vi "E725_Simple_Test.vi"(0 "System no.":i32=1 min=1 max=4 step=1, 2 "Interface":u16(ring) items=["RS232", "TCP/IP", "USB"], 3 "Timeout":u32=5000, 5 "error in":errorcluster, 6 "RS232 settings":cluster{"Portnumber":u16, "Baudrate":u16}={"Portnumber"=0, "Baudrate"=5} {"Baudrate" items=["9600", "14400", "19200", "38400", "57600", "115200"]; "Portnumber" items=["COM1", "COM2", "COM3", "COM4", "COM5", "COM6", "COM7", "COM8", "COM9"]}, 7 "TCP/IP settings":T1={"Host address/name"="localhost", "Port"=50000, "Board"=0, "TCP/IP Search?"=TRUE}, 8 "USB settings":cluster{"S/N":string, "USB Search?":bool}={"S/N"="", "USB Search?"=TRUE}) -> (14 "Identification":string, 15 "Helpstring":string, 16 "Conn. Axes":string[](array[string]), 17 "Position":dbl[](array[numeric]) format="%.6f", 19 "error out":errorcluster)   [LabVIEW 2009]
doc: "This simple test VI is a stand-alone sample application. Use the Help?Show Context Help menu sequence in the LabVIEW environment to display the Context Help window with the VI and control/indicator descriptions.\n\nSpecify \n¢ System no. (= 1 in a one-system configuration),\n¢ Interface (= RS232, TCP/IP or USB)\n¢ Timeout value (in milliseconds)\n¢ and interface settings first.\n\nThen start the VI. The VI will open a connection to the E-712 and query the controller for its identification string (*IDN?), help string (HLP?), the IDs (SAI?) and stage names (CST?) of the connected axes and their current position values (POS?). The diagram shows how to combine the driver and support VIs for these tasks."
panel:
  out "Stage names":string[](array[string])
  # "Simple E-712 communication test program"
  # "Select E-712 interface, timeout value and interface settings first, then start the VI. \nThe VI will open the chosen port, query for the connected axes (SAI?), the stage names (SAI?), the position (POS?), Identification (*IDN?) and help string\n(HLP?). See VI and control/ indicator information for details."
  # "Only for\nInterface = \nTCP/IP:"
  # "Only for\nInterface = \nRS232:"
  # "Only for\nInterface = \nUSB:"
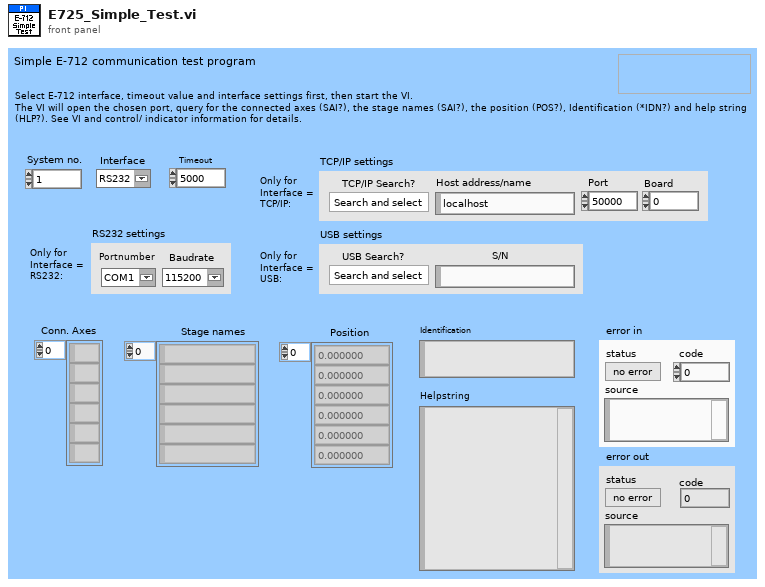
[diagram p1: front panel]
types:
  T1 = cluster{"Host address/name":string, "Port":i32, "Board":i32, "TCP/IP Search?":bool}
  T2 = cluster{"Host address/name":string, "Port":i32, "Board":i32}
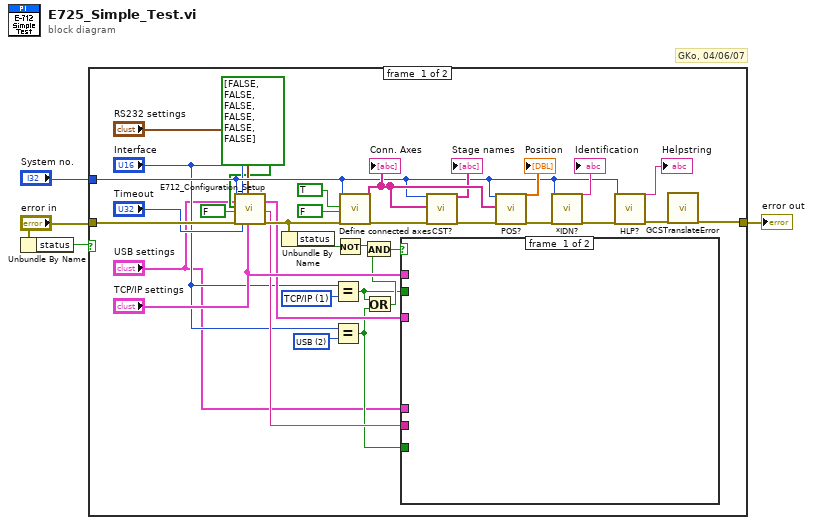
[diagram p0: block diagram]
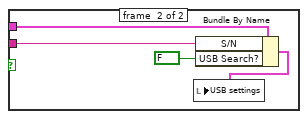
[diagram p3: hidden frame]
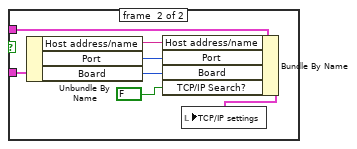
[diagram p4: hidden frame]
diagram:
  # "GKo, 04/06/07"
  n1 = Unbundle By Name("error in") -> ("status"=w2:bool)
  n2 = case shown="False" w2 {
    tunnel: [w37 w55] -> w3
    tunnel: "error in" -> [w24 w55]
    tunnel: "System no." -> [w23 _]
    frame #0 {
      w10 = u16 2 items=["RS232", "TCP/IP", "USB"] ("Interface")
      w11 = u16 1 items=["RS232", "TCP/IP", "USB"] ("Interface")
      n3 = call "E712_Configuration_Setup.vi"("System no."=w23, "USB settings"="USB settings", "Are stages connected?"=bool[] [FALSE, FALSE, FALSE, FALSE, FALSE, FALSE], "Change servo status to ON?"=FALSE ("Connected?"), "error in"=w24, "Interface"="Interface", "Timeout"="Timeout", "RS232 settings"="RS232 settings", "TCP/IP settings"="TCP/IP settings") -> ("TCP/IP settings out"=w14:T2, "USB: S/N out"=w13:string, "error out"=w19:errorcluster)  [unwired: 6 in, 2 out]
      n4 = Unbundle By Name(w19) -> ("status"=w18:bool)
      n5 = Equal?(x="Interface", y=w11) -> (x = y?=w8:bool)
      n6 = Equal?(x="Interface", y=w10) -> (x = y?=w7:bool)
      n7 = Not(x=w18) -> (.not. x?=w16:bool)
      n8 = call "Define connected axes.vi"("System no."=w23, "Read from\ncontroller?"=TRUE ("Read from\nController"), "Invert\norder?"=FALSE ("Invert\nOrder"), "error in"=w19) -> ("Conn. Axes out"=w26:string[], "error out"=w28:errorcluster)  [unwired: 14 in]
      "Conn. Axes" <- w26
      n9 = Or(x=w8, y=w7) -> (x .or. y?=w9:bool)
      n10 = And(x=w16, y=w9) -> (x .and. y?=w17:bool)
      n11 = case shown="True" w17 {
        tunnel: "TCP/IP settings" -> [_ w43]
        tunnel: w14 -> [_ w42]
        tunnel: w13 -> [_ w40]
        tunnel: "USB settings" -> [_ w41]
        tunnel: w8 -> [_ w39]
        tunnel: w7 -> [_ w38]
        frame #0 {
        }
        frame #1 {
          n12 = case shown="True" w39 {
            tunnel: w43 -> [_ w53]
            tunnel: w42 -> [_ w51]
            frame #0 {
            }
            frame #1 {
              n13 = Unbundle By Name(w51) -> ("Host address/name"=w50:string, "Port"=w49:i32, "Board"=w48:i32)
              n14 = Bundle By Name(cluster=w53, "Host address/name"=w50, "Port"=w49, "Board"=w48, "TCP/IP Search?"=FALSE) -> (w54:T1)
              n15 = local write "TCP/IP settings"(w54) -> ()
            }
          }
          n16 = case shown="True" w38 {
            tunnel: w41 -> [_ w47]
            tunnel: w40 -> [_ w45]
            frame #0 {
            }
            frame #1 {
              n17 = Bundle By Name(cluster=w47, "S/N"=w45, "USB Search?"=FALSE ("TCP/IP Search?")) -> (w44:cluster{"S/N":string, "USB Search?":bool})
              n18 = local write "USB settings"(w44) -> ()
            }
          }
        }
      }
      n19 = call "CST?.vi"("System no."=w23, "Axes to query"=w26, "error in"=w28) -> ("Stage names"=→"Stage names":string[], "error out"=w27:errorcluster)  [unwired: 15 in]
      n20 = call "POS?.vi"("System no."=w23, "Axes to query"=w26, "error in"=w27) -> ("Position"=→"Position":dbl[], "error out"=w30:errorcluster)  [unwired: 15 in]
      n21 = call "*IDN?.vi"("System no."=w23, "error in"=w30) -> ("Identification"=→"Identification":string, "error out"=w36:errorcluster)  [unwired: 16 in]
      n22 = call "HLP?.vi"("System no."=w23, "error in"=w36) -> ("Help string"=→"Helpstring":string, "error out"=w29:errorcluster)  [unwired: 16 in]
      n23 = call "GCSTranslateError.vi"("error in"=w29) -> ("error out"=w37:errorcluster)  [unwired: 16 in, 2 out]
    }
    frame #1 {
    }
  }
  "error out" <- w3
